vi "SIM.vi"() -> ()   [LabVIEW 2013]
panel:
  out "PotPosOut":dbl
  out "IsThere":bool
  out "CamPow":dbl
  out "CamPosOut":dbl
  in  "FireButton":bool
  in  "three":bool
  in  "two":bool
  in  "one":bool
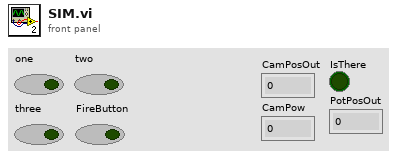
[diagram p1: front panel]
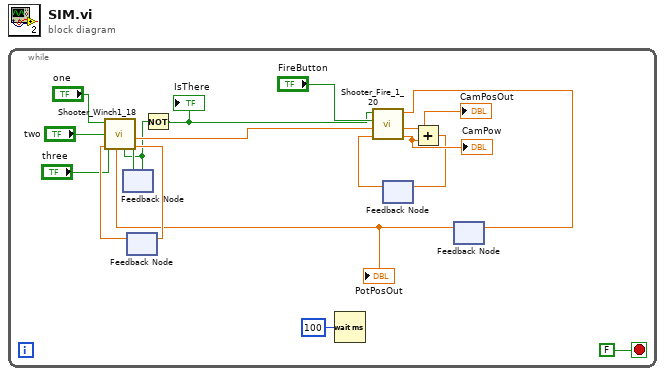
[diagram p0: block diagram]
diagram:
  n1 = while {
    stop <- FALSE stop-if-true
    n2 = feedback #1() -> (w1:bool)  [unwired: 1 in]
    n3 = feedback #2() -> (w15:dbl)  [unwired: 1 in]
    n4 = Not(x=w1) -> (.not. x?=w6:bool)
    "IsThere" <- w6
    n5 = Wait (ms)(milliseconds to wait=u32 100) -> ()  [unwired: 1 out]
    n6 = feedback #3() -> (w7:dbl)  [unwired: 1 in]
    n7 = feedback #4() -> (w3:dbl)  [unwired: 1 in]
    "PotPosOut" <- w3
    n8 = call "Shooter_Winch1_18.vi"("IsNotThereIn"=w1, "Winch Pot Location"=w3, "LastIndex"=w15, "three"="three", "two"="two", "one"="one") -> ("LastIndexOut"=w16:dbl, "Winch Pot LocationOut"=w5:dbl, "IsNotThere"=w2:bool)  [unwired: 3 in]
    n9 = feedback-in #1(w2) -> ()
    n10 = feedback-in #2(w16) -> ()
    n11 = call "Shooter_Fire_1_20.vi"("CamPos"=w7, "PotPos In"=w5, "FireButton"="FireButton", "IsReady"=w6) -> ("CamPow"=w9:dbl, "CamPosOut"=w10:dbl, "PotPosOut"=w4:dbl)  [unwired: 5 in]
    "CamPosOut" <- w10
    "CamPow" <- w9
    n12 = Add(x=w10, y=w9) -> (x+y=w8:dbl)
    n13 = feedback-in #3(w8) -> ()
    n14 = feedback-in #4(w4) -> ()
  }
